vi "AvoidWall.vi"(3 "SupressIn":dbl, 7 "Inhibit":bool, 8 "HowAmI? Clean":cluster{"T":dbl, "Battery":dbl, "Temp":dbl}, 9 "WhatAroundMe? Clean":cluster{"T":dbl, "Range":dbl, "Bearing":dbl}[](array[cluster]), 11 "Velocity":dbl) -> (0 "SupressOut":dbl, 2 "ActCommand":dbl[](array[numeric]), 10 "Boat":T1)   [LabVIEW 2011]
doc: "This subVI behavior avoids walls parallel to teh direction of the robot. It does so by finding the centroid of the LIDAR data if the robot is within 20 pixels of the wall and placing a noraml distribution at that point.\n\nIt is designed to work with a 90 element behavior arbiter."
uses:
  WhereAmI.ctl
  <vilib>/Analysis/2dsp.llb/Integral Method.ctl
  <vilib>/Analysis/1siggen.llb/Ramp Pattern by Samples.vi
  <vilib>/Analysis/8numeric.llb/1D Numeric Integration.vi
  <vilib>/gmath/statdist.llb/Normal PDF.vi
  <vilib>/Analysis/NI_AALPro.lvlib
  <vilib>/gmath/NI_Gmath.lvlib
  <vilib>/Analysis/NI_AALBase.lvlib
panel:
  out "x+y":dbl
  out "Waveform Graph":dbl[][](graph)
  # "This contains a behavior that steers away from walls when they are too close"
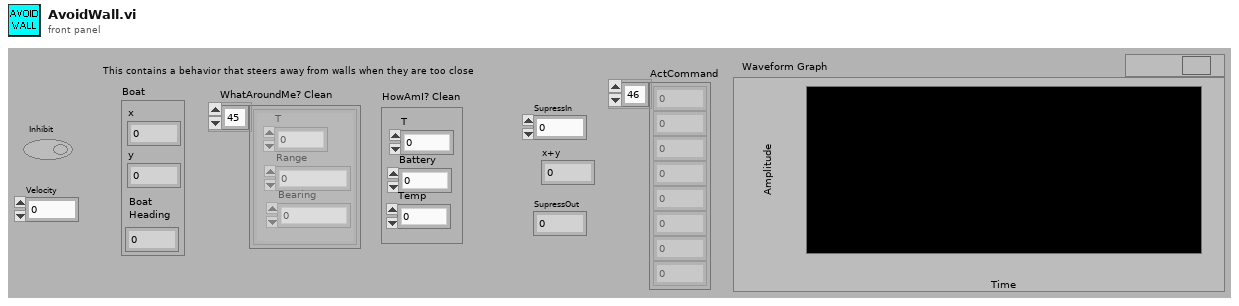
[diagram p1: front panel]
types:
  T1 = typedef "WhereAmI.ctl" = cluster{"x":sgl, "y":sgl, "Boat\nHeading":sgl}
  T2 = typedef "NI_AALPro.lvlib/Integral Method.ctl" = i32
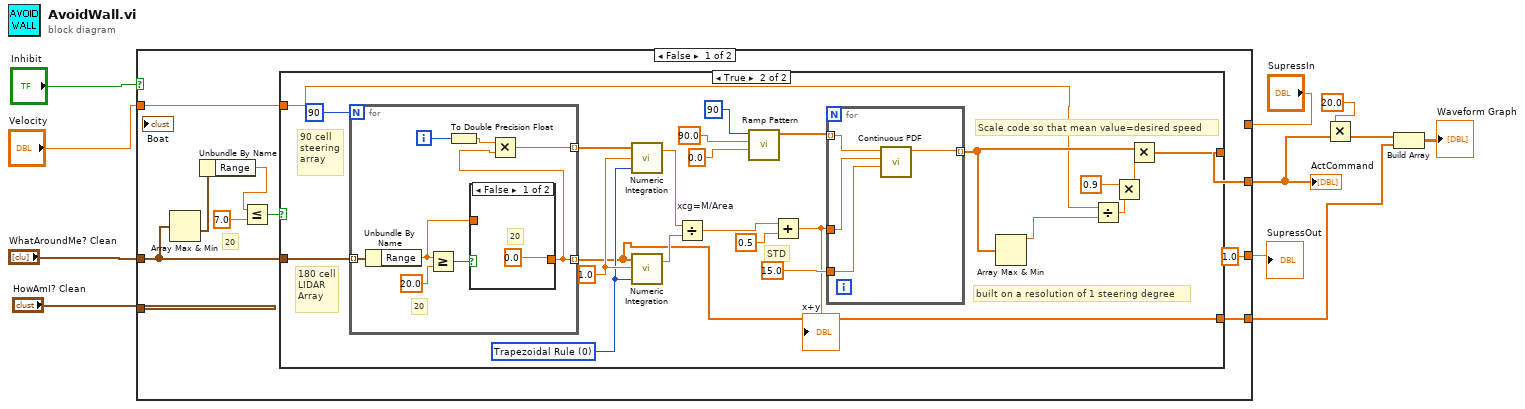
[diagram p0: block diagram]
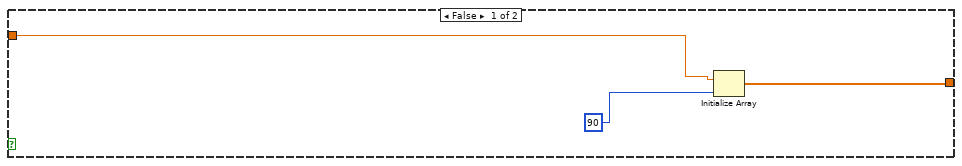
[diagram p2: hidden frame]
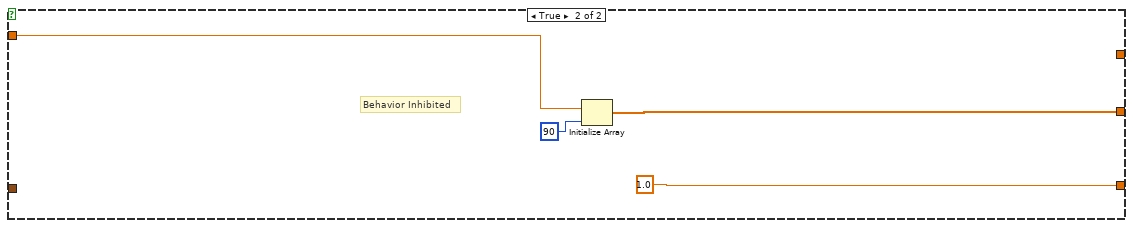
[diagram p4: hidden frame]
diagram:
  n1 = case shown="False" "Inhibit" {
    tunnel: "Velocity" -> [w18 w61]
    tunnel: "WhatAroundMe? Clean" -> [w16 _]
    tunnel: "HowAmI? Clean" -> [_ _]
    tunnel: "SupressIn" -> [_ _]
    tunnel: [w19 w62] -> w5
    tunnel: [1.0 ("SupressOut") 1.0 ("SupressOut")] -> w6
    tunnel: [w17 _] -> w3
    frame False {
      # "20"
      n2 = Array Max & Min(array=w16) -> (min value=w15:cluster{"T":dbl, "Range":dbl, "Bearing":dbl})  [unwired: 3 out]
      n3 = Unbundle By Name(w15) -> ("Range"=w13:dbl)
      n4 = Less Or Equal?(x=w13, y=7.0) -> (x <= y?=w14:bool)
      n5 = case shown="True" w14 {
        tunnel: w16 -> [_ w45]
        tunnel: [w22 w33] -> w19
        tunnel: w18 -> [w21 w31]
        tunnel: [_ w27] -> w17
        frame False {
          n6 = Initialize Array "Initialize Array"(w21, 90 ("dimension size")) -> (w22:dbl[])
        }
        frame True {
          w43 = 1.0 ("dt")
          w42 = T2 0 items=["Trapezoidal Rule", "Simpson's Rule", "Simpson's 3/8 Rule", "Bode Rule"] ("integration method")
          # "built on a resolution of 1 steering degree"
          # "Scale code so that mean value=desired speed"
          # "STD"
          # "180 cell\nLIDAR \nArray"
          # "90 cell\nsteering\narray"
          n7 = for {
            N: 90 -> [_]
            tunnel: w45 -> [w58] mode=indexing
            tunnel: [w53] -> w27 mode=indexing
            tunnel: [w51] -> w44 mode=indexing
            i -> [w54]
            # "20"
            n8 = Unbundle By Name(w58) -> ("Range"=w55:dbl)
            n9 = Greater Or Equal?(x=w55, y=20.0) -> (x >= y?=w56:bool)
            n10 = To Double Precision Float(number=w54) -> (double precision float=w52:dbl)
            n11 = case shown="False" w56 {
              tunnel: w55 -> [_ w60]
              tunnel: [0.0 ("Range") w60] -> w53
              frame False {
                # "20"
              }
              frame True {
              }
            }
            n12 = Multiply(x=w52, y=w53) -> (x*y=w51:dbl)
          }
          n13 = call-poly <vilib>:"Numeric Integration.vi"("integration method"=w42, "dt"=w43, "Input Array"=w44) -> ("result"=w32:dbl)  [unwired: 1 out]
          n14 = call-poly <vilib>:"Numeric Integration.vi"("integration method"=w42, "dt"=w43, "Input Array"=w27) -> ("result"=w41:dbl)  [unwired: 1 out]
          n15 = Divide "xcg=M/Area"(x=w32, y=w41) -> (x/y=w30:dbl)
          n16 = call-poly <vilib>:"Ramp Pattern.vi"("start"=0.0, "end"=90.0 ("end (Normal)"), "samples"=90) -> ("Ramp Pattern"=w26:dbl[])  [unwired: 7 in, 1 out]
          n17 = Add(x=w30, y=0.5) -> (x+y=w29:dbl)
          "x+y" <- w29
          n18 = for {
            tunnel: w26 -> [w50] mode=indexing
            tunnel: 15.0 ("std (Normal)") -> [w49]
            tunnel: [w48] -> w39 mode=indexing
            tunnel: w29 -> [w47]
            n19 = call-poly <vilib>:"Continuous PDF.vi"("std"=w49, "mean"=w47, "x"=w50) -> ("pdf(x)"=w48:dbl)  [unwired: 7 in, 1 out]
          }
          n20 = Array Max & Min(array=w39) -> (max value=w37:dbl)  [unwired: 3 out]
          n21 = Divide(x=w31, y=w37) -> (x/y=w38:dbl)
          n22 = Multiply(x=0.9, y=w38) -> (x*y=w25:dbl)
          n23 = Multiply(x=w39, y=w25) -> (x*y=w33:dbl[])
        }
      }
    }
    frame True {
      # "Behavior Inhibited"
      n24 = Initialize Array "Initialize Array"(w61, 90 ("dimension size")) -> (w62:dbl[])
    }
  }
  "ActCommand" <- w5
  "SupressOut" <- w6
  n25 = Multiply(x=20.0, y=w5) -> (x*y=w2:dbl[])
  n26 = Build Array(w2, w3) -> (→"Waveform Graph":dbl[][])
